vi "Write Data Labels to file.vi"(8 "error in":errorcluster, 11 "Report Generator in":refnum<class "Report Generator.lvclass">) -> (0 "error out":errorcluster, 3 "Report Generator out":refnum<class "Report Generator.lvclass">)   [LabVIEW 2018, in "Report Generator.lvlib" / "Report Generator.lvclass"]
uses:
  Report Generator.lvclass
  Report Generator.lvclass/Report Generator.ctl
  <vilib>/Utility/file.llb/Write Delimited Spreadsheet (string).vi
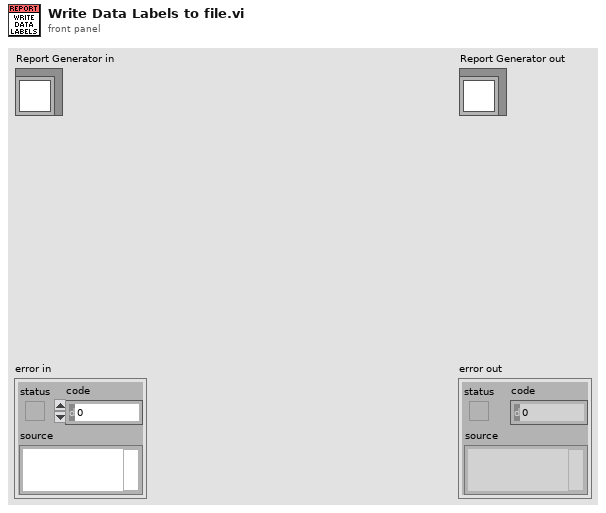
[diagram p1: front panel]
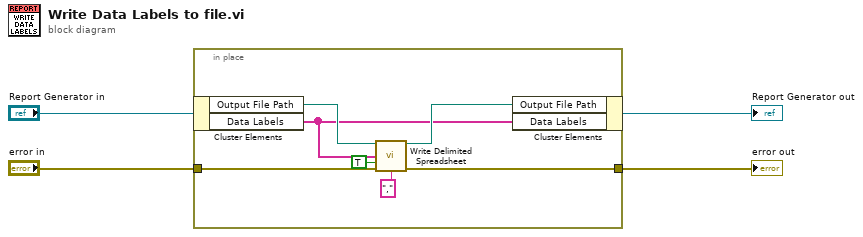
[diagram p0: block diagram]
diagram:
  n1 = in-place {
    in-place-border: [w7] -> w2
    in-place-border: "error in" -> [w5]
    n2 = in-place-cluster #1("Report Generator in") -> ("Output File Path"=w11:path, "Data Labels"=w8:string[])
    n3 = call-poly <vilib>:"Write Delimited Spreadsheet.vi"("file path (dialog if empty)"=w11, "1D data"=w8, "append to file? (new file:F)"=TRUE, "error in (no error)"=w5, "delimiter (\\t)"="," ("delimiter (\\t)")) -> ("new file path (Not A Path if cancelled)"=w10:path, "error out"=w7:errorcluster)  [unwired: 9 in]
    n4 = in-place-cluster #1("Output File Path"=w10, "Data Labels"=w8) -> (→"Report Generator out":refnum<class "Report Generator.lvclass">)
  }
  "error out" <- w2
